vi "Page_Source_Settings_CustVISettings_UpdateDisplay.vi"(8 "error in (no error)":errorcluster, 9 "sourceInclusion":T1, 10 "sourceProperties in":T2[](array[typedef]), 11 "AB_Application in":refnum<class "AB_Application.lvclass">) -> (0 "error out":errorcluster, 1 "Run when opened disabled state":u8, 2 "sourceProperties out":T2[](array[typedef]), 3 "AB_Application out":refnum<class "AB_Application.lvclass">, 5 "AEH disabled state":u8)   [LabVIEW 2020, in "AB_Application.lvclass"]
uses:
  <vilib>/AppBuilder/AB_Classes/Application/AB_Application.lvclass
  <vilib>/AppBuilder/AB_Source_Properties.ctl
  <vilib>/AppBuilder/AB_Source_Property_Type.ctl
  <vilib>/AppBuilder/AB_Source_Inclusion.ctl
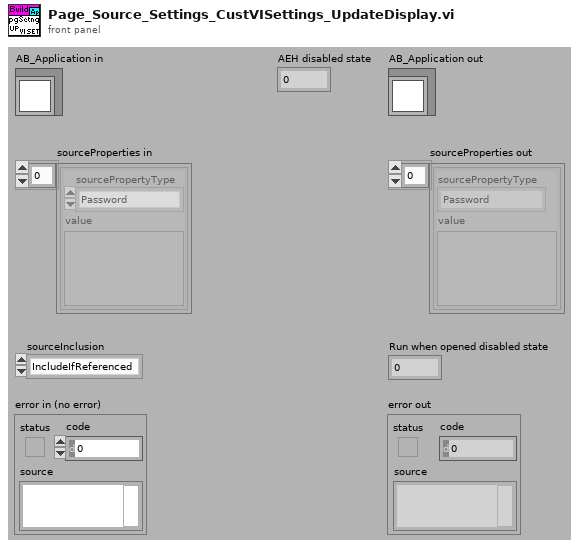
[diagram p1: front panel]
types:
  T1 = typedef "AB_Source_Inclusion.ctl" = enum16{"IncludeIfReferenced", "Include", "Exclude", "TopLevel"}
  T2 = typedef "AB_Source_Properties.ctl" = cluster{"sourcePropertyType":T3, "value":variant}
  T3 = typedef "AB_Source_Property_Type.ctl" = enum16{"Remove block diagram", "Remove front panel", "Password", "Window has title bar", "Show menu bar", "Show vertical scroll bar", "Show horizontal scroll bar", "Show toolbar", "Show Abort button", "Show fp when called", "Window behavior", "Allow user to close window", "Window run-time position", "Run when opened", "Allow debugging", "Auto error handling", "Generate guard code", "Use stack variables", "Expression folding", "Integer only", "Inline subVI"}
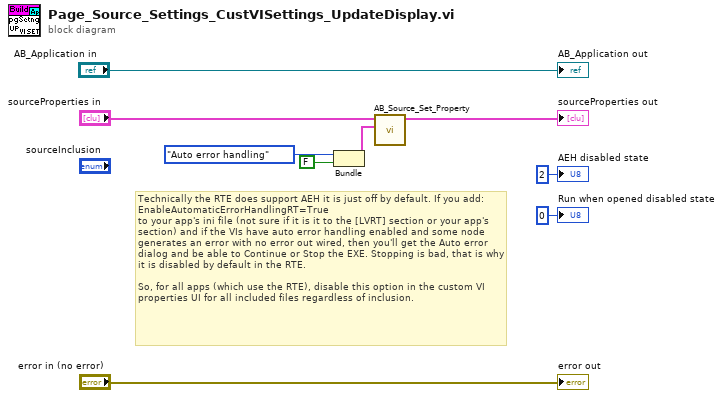
[diagram p0: block diagram]
diagram:
  # "Technically the RTE does support AEH it is just off by default. If you add: EnableAutomaticErrorHandlingRT=True\nto your app's ini file (not sure if it is it to the [LVRT] section or your app's section) and if the VIs have auto error handling enabled and some node generates an error with no error out wired, then you'll get the Auto error dialog and be able to Continue or Stop the EXE. Stopping is bad, that is why it is disabled by default in the RTE.\n\nSo, for all apps (which use the RTE), disable this option in the custom VI properties UI for all included files regardless of inclusion."
  n1 = Bundle("type"=AB_Source_Property_Type."Auto error handling", FALSE) -> (w6:cluster{"type":T3, bool})  [unwired: 1 in]
  n2 = call <vilib>:"AB_Source_Set_Property.vi"("sourceProperty"=w6, "sourceProperties in"="sourceProperties in") -> ("sourceProperties out"=→"sourceProperties out":T2[])  [unwired: 7 in, 2 out]
  "error out" <- "error in (no error)"
  "AB_Application out" <- "AB_Application in"
  "Run when opened disabled state" <- u8 0 ("Run when opened disabled state")
  "AEH disabled state" <- u8 2 ("AEH disabled state")
